vi "Close control references.vi"(8 "Error In":errorcluster, 11 "UI Data":T1) -> (0 "Error Out":errorcluster, 3 "UI Data Out":T1)   [LabVIEW 2015]
doc: "VI closes and controls references."
uses:
  controls/UI Data.ctl
  controls/Instruments.ctl
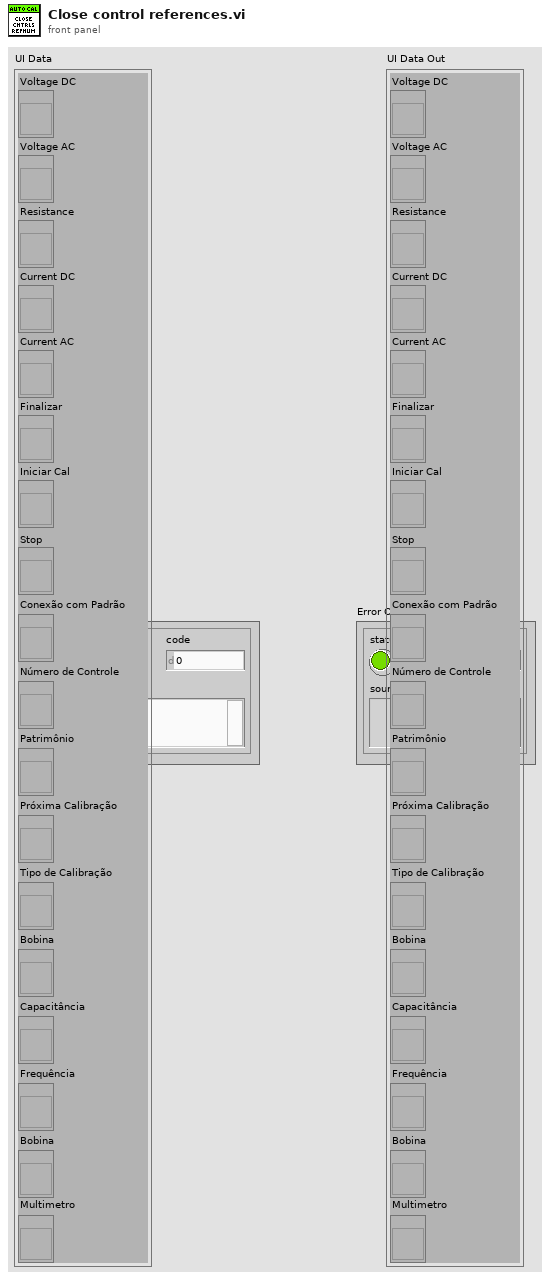
[diagram p1: front panel]
types:
  T1 = typedef "UI Data.ctl" = cluster{"Voltage DC":refnum<vi>, "Voltage AC":refnum<vi>, "Resistance":refnum<vi>, "Current DC":refnum<vi>, "Current AC":refnum<vi>, "Finalizar":refnum<vi>, "Iniciar Cal":refnum<vi>, "Stop":refnum<vi>, "Conexão com Padrão":refnum<vi>, "Número de Controle":refnum<vi>, "Patrimônio":refnum<vi>, "Próxima Calibração":refnum<vi>, "Tipo de Calibração":refnum<vi>, "Bobina":refnum<vi>, "Capacitância":refnum<vi>, "Frequência":refnum<vi>, "Bobina":refnum<vi>, "Multimetro":refnum<vi>}
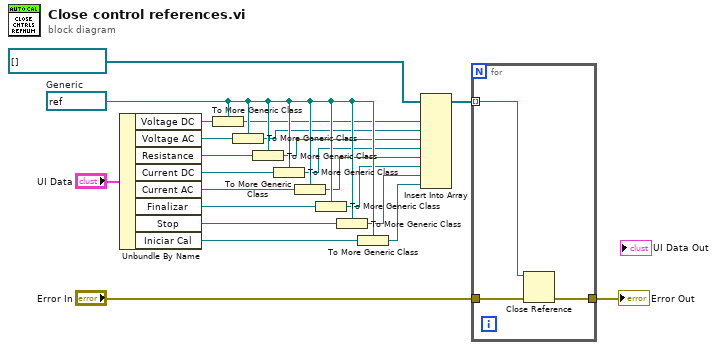
[diagram p0: block diagram]
diagram:
  w15 = refnum<vi> refnum  # Generic
  n1 = Unbundle By Name("UI Data") -> ("Voltage DC"=w19:refnum<vi>, "Voltage AC"=w18:refnum<vi>, "Resistance"=w17:refnum<vi>, "Current DC"=w16:refnum<vi>, "Current AC"=w13:refnum<vi>, "Finalizar"=w12:refnum<vi>, "Stop"=w11:refnum<vi>, "Iniciar Cal"=w14:refnum<vi>)
  n2 = To More Generic Class(target class=w15, reference=w19) -> (generic class reference=w9:refnum<vi>)
  n3 = To More Generic Class(target class=w15, reference=w18) -> (generic class reference=w8:refnum<vi>)
  n4 = To More Generic Class(target class=w15, reference=w17) -> (generic class reference=w7:refnum<vi>)
  n5 = To More Generic Class(target class=w15, reference=w16) -> (generic class reference=w6:refnum<vi>)
  n6 = To More Generic Class(target class=w15, reference=w13) -> (generic class reference=w5:refnum<vi>)
  n7 = To More Generic Class(target class=w15, reference=w12) -> (generic class reference=w4:refnum<vi>)
  n8 = To More Generic Class(target class=w15, reference=w11) -> (generic class reference=w3:refnum<vi>)
  n9 = To More Generic Class(target class=w15, reference=w14) -> (generic class reference=w2:refnum<vi>)
  n10 = Insert Into Array(array=refnum<vi>[] [], new element #1=w9, new element #2=w8, new element #3=w7, new element #4=w6, new element #5=w5, new element #6=w4, new element #7=w3, new element #8=w2) -> (w1:refnum<vi>[])  [unwired: 1 in]
  n11 = for {
    tunnel: w1 -> [w24] mode=indexing
    tunnel: "Error In" -> [w25]
    tunnel: [w23] -> w21
    n12 = Close Reference(reference=w24, error in (no error)=w25) -> (error out=w23:errorcluster)
  }
  "Error Out" <- w21
